vi "VToutput.vi"(10 "Elapsed Time (s)":dbl, 11 "Length set point [mm]":dbl) -> (3 "V":dbl)   [LabVIEW 2013]
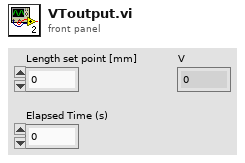
[diagram p1: front panel]
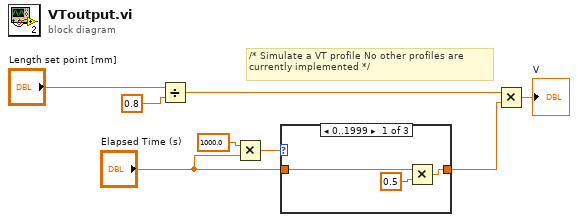
[diagram p0: block diagram]
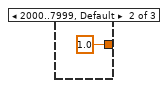
[diagram p2: hidden frame]
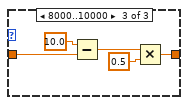
[diagram p3: hidden frame]
diagram:
  # "/* Simulate a VT profile No other profiles are currently implemented */"
  n1 = Divide(x="Length set point [mm]", y=0.8 ("Setpoint")) -> (x/y=w2:dbl)
  n2 = Multiply(x=1000.0, y="Elapsed Time (s)") -> (x*y=w4:dbl)
  n3 = case shown="0..1999" w4 {
    tunnel: "Elapsed Time (s)" -> [w11 _ w14]
    tunnel: [w9 1.0 ("y") w16] -> w1
    frame 0..1999 {
      n4 = Multiply(x=w11, y=0.5) -> (x*y=w9:dbl)
    }
    frame 2000..7999, Default {
    }
    frame 8000..10000 {
      n5 = Subtract(x=10.0, y=w14) -> (x-y=w15:dbl)
      n6 = Multiply(x=w15, y=0.5) -> (x*y=w16:dbl)
    }
  }
  n7 = Multiply(x=w2, y=w1) -> (x*y=→"V":dbl)
